vi "MGI Calculate Peak Moments.vi"(3 "Width (0: whole array)":i32, 4 "Start Index (0)":i32, 5 "Signal[]":dbl[](array[numeric]) format="%.2f") -> (0 "RMS Peak Width":dbl format="%.2e", 1 "Peak Centroid":dbl format="%.2f", 2 "Peak Area":dbl format="%.2e")   [LabVIEW 2016]
doc: "Calculate peak moments for an evenly sampled signal.\n0th moment is the area under the peak i.e. the sum of the signals\n1st moment is the location of the peak/centroid/center of mass. Calculated by sum(i*yi)/sum(yi), it's in units of the spacing between the signals, with 0 corresponding to the first element of the array.\n2nd moment is the RMS peak width, also in index units.\n\nAuthored by David A. Moore\nsupport@mooregoodideas.com\nwww.mooregoodideas.com\n\nCopyright (c) 2010, Moore Good Ideas, Inc.\n\nAll rights reserved.\n\nRedistribution and use in source and binary forms, with or without modification, are permitted provided that the following conditions are met:\n\n * Redistributions of source code must retain the above copyright notice, this list of conditions and the following disclaimer.\n * Redistributions in binary form must reproduce the above copyright notice, this list of conditions and the following disclaimer in the documentation and/or other materials provided with the distribution.\n * Neither the name of Moore Good Ideas, Inc. nor the names of its contributors may be used to endorse or promote products derived from this software without specific prior written permission.\n\nTHIS SOFTWARE IS PROVIDED BY THE COPYRIGHT HOLDERS AND CONTRIBUTORS \"AS IS\" AND ANY EXPRESS OR IMPLIED WARRANTIES, INCLUDING, BUT NOT LIMITED TO, THE IMPLIED WARRANTIES OF MERCHANTABILITY AND FITNESS FOR A PARTICULAR PURPOSE ARE DISCLAIMED. IN NO EVENT SHALL THE COPYRIGHT OWNER OR CONTRIBUTORS BE LIABLE FOR ANY DIRECT, INDIRECT, INCIDENTAL, SPECIAL, EXEMPLARY, OR CONSEQUENTIAL DAMAGES (INCLUDING, BUT NOT LIMITED TO, PROCUREMENT OF SUBSTITUTE GOODS OR SERVICES; LOSS OF USE, DATA, OR PROFITS; OR BUSINESS INTERRUPTION) HOWEVER CAUSED AND ON ANY THEORY OF LIABILITY, WHETHER IN CONTRACT, STRICT LIABILITY, OR TORT (INCLUDING NEGLIGENCE OR OTHERWISE) ARISING IN ANY WAY OUT OF THE USE OF THIS SOFTWARE, EVEN IF ADVISED OF THE POSSIBILITY OF SUCH DAMAGE."
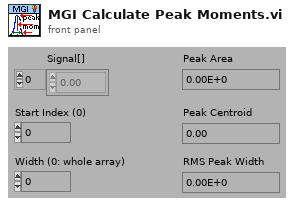
[diagram p1: front panel]
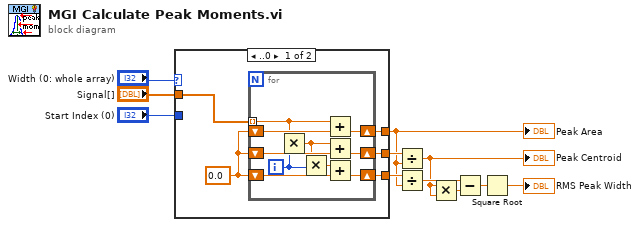
[diagram p0: block diagram]
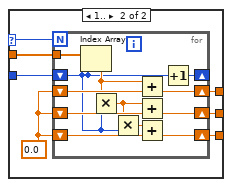
[diagram p2: hidden frame]
diagram:
  n1 = case shown="..0" "Width (0: whole array)" {
    selector: "Width (0: whole array)" -> [_ w28]
    tunnel: "Signal[]" -> [w16 w33]
    tunnel: [w14 w31] -> w10
    tunnel: [w13 w30] -> w9
    tunnel: [w12 w29] -> w8
    tunnel: "Start Index (0)" -> [_ w27]
    frame ..0 {
      w15 = 0.0
      n2 = for {
        tunnel: w16 -> [w24] mode=indexing
        shift-right: [w25] -> w12
        shift-left: w15 -> [w26]
        shift-right: [w22] -> w14
        shift-left: w15 -> [w23]
        shift-right: [w18] -> w13
        shift-left: w15 -> [w17]
        i -> [w20]
        n3 = Multiply(x=w24, y=w20) -> (x*y=w21:dbl)
        n4 = Multiply(x=w21, y=w20) -> (x*y=w19:dbl)
        n5 = Add(x=w24, y=w26) -> (x+y=w25:dbl)
        n6 = Add(x=w21, y=w23) -> (x+y=w22:dbl)
        n7 = Add(x=w19, y=w17) -> (x+y=w18:dbl)
      }
    }
    frame 1.. {
      w32 = 0.0
      n8 = for {
        N: w28 -> [_]
        tunnel: w33 -> [w35]
        shift-right: [w44] -> w29
        shift-left: w32 -> [w45]
        shift-right: [w42] -> w31
        shift-left: w32 -> [w43]
        shift-right: [w39] -> w30
        shift-left: w32 -> [w38]
        shift-right: [w37] -> _
        shift-left: w27 -> [w34]
        n9 = Index Array(array=w35, index=w34) -> (element=w36:dbl)
        n10 = Multiply(x=w36, y=w34) -> (x*y=w41:dbl)
        n11 = Multiply(x=w41, y=w34) -> (x*y=w40:dbl)
        n12 = Add(x=w36, y=w45) -> (x+y=w44:dbl)
        n13 = Add(x=w41, y=w43) -> (x+y=w42:dbl)
        n14 = Add(x=w40, y=w38) -> (x+y=w39:dbl)
        n15 = Increment(x=w34) -> (x+1=w37:i32)
      }
    }
  }
  "Peak Area" <- w8
  n16 = Divide(x=w10, y=w8) -> (x/y=w5:dbl)
  "Peak Centroid" <- w5
  n17 = Divide(x=w9, y=w8) -> (x/y=w7:dbl)
  n18 = Multiply(x=w5, y=w5) -> (x*y=w6:dbl)
  n19 = Subtract(x=w7, y=w6) -> (x-y=w4:dbl)
  n20 = Square Root(x=w4) -> (sqrt(x)=→"RMS Peak Width":dbl)
